vi "OpenCVFaceDetection_NewMat.vi"(8 "ErrorIn":errorcluster, 10 "CmdData":variant, 11 "OpenCVFaceDetectionIn":refnum<class>) -> (0 "ErrorOut":errorcluster, 2 "ReplyData":variant, 3 "OpenCVFaceDetectionOut":refnum<class>, 4 "Exit":bool)   [LabVIEW 2021, in "OpenCVFaceDetection.lvclass"]
uses:
  OpenCVFaceDetection.lvclass
  OpenCVFaceDetection_UiCallBackEvents.ctl
  OpenCVFaceDetection.lvclass/OpenCVFaceDetection.ctl
  9f33c80a-1a62-43e8-9ad8-ec198e7f1f80.vi
  System.Drawing
  C:/Localdata/Projects/TriekselSoft/TriekselsoftApplicationFramework/Source/.Externals/Library_EmguCV/Emgu.CV.Platform.NetStandard.dll
  .Externals/Library_EmguCV/Emgu.CV.Platform.NetStandard.dll
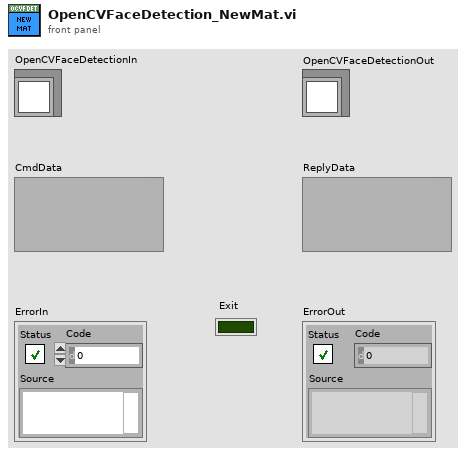
[diagram p1: front panel]
types:
  T1 = typedef "OpenCVFaceDetection.lvclass/OpenCVFaceDetection_UiCallBackEvents.ctl" = enum16{"Default", "PersistentDataUpdated", "NewPicture", "Worker 1: Do Something"}
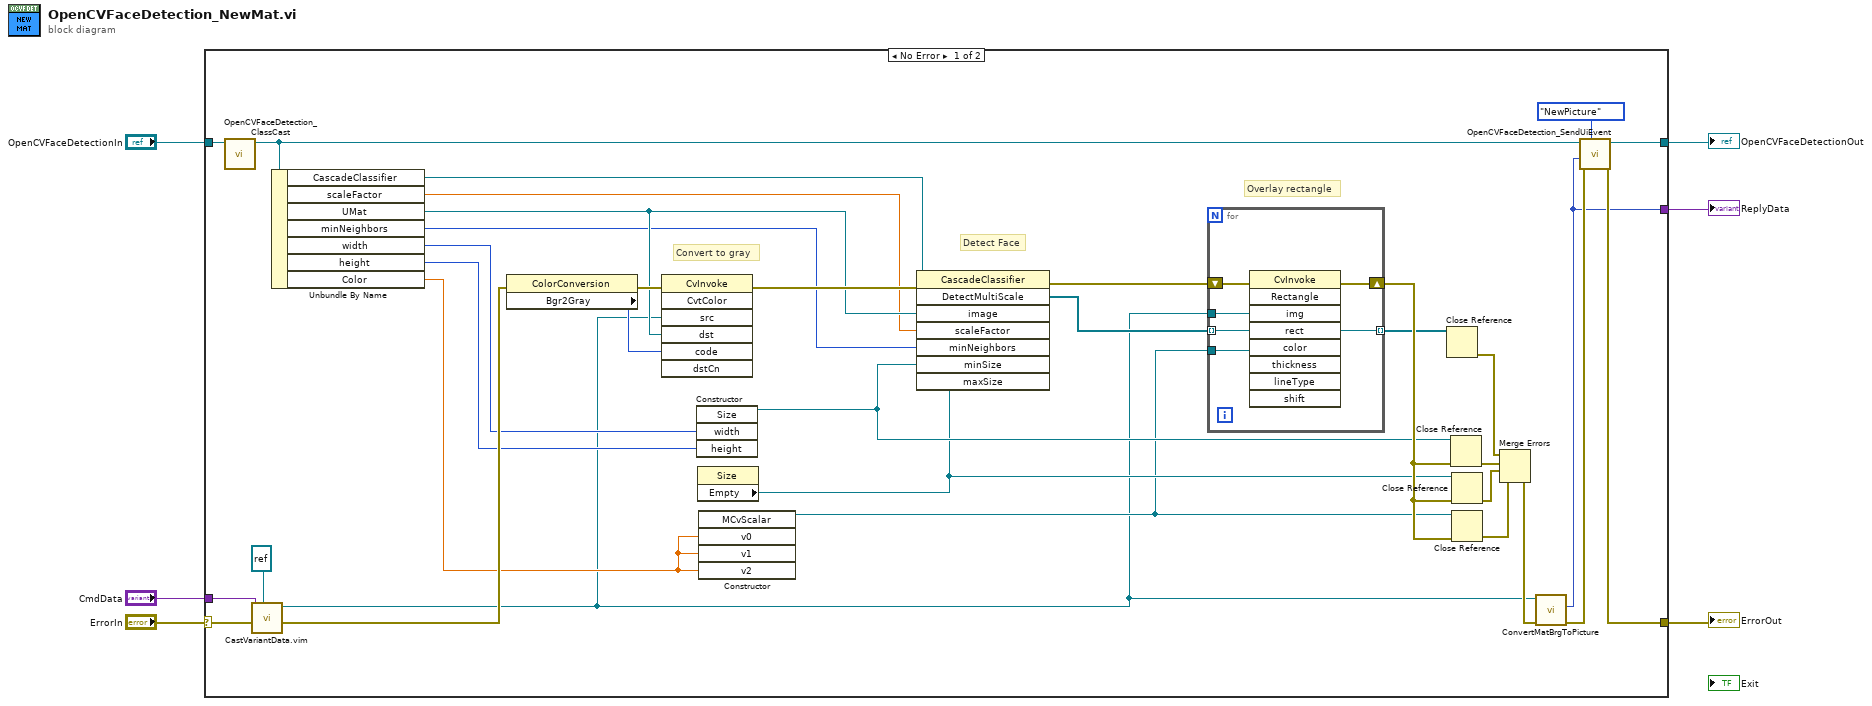
[diagram p0: block diagram]
diagram:
  n1 = case shown="No Error" "ErrorIn" {
    selector: "ErrorIn" -> [w40 w48]
    tunnel: [w29 w48] -> w5
    tunnel: [w9 w47] -> w3
    tunnel: "CmdData" -> [w26 w47]
    tunnel: "OpenCVFaceDetectionIn" -> [w27 w46]
    tunnel: [w10 w46] -> w1
    frame No Error {
      # "Overlay rectangle"
      # "Detect Face"
      # "Convert to gray"
      n2 = call "OpenCVFaceDetection_ClassCast.vi"("OpenCVFaceDetectionIn"=w27) -> ("OpenCVFaceDetectionOut"=w20:refnum<class "OpenCVFaceDetection.lvclass">)  [unwired: 10 in]
      n3 = call "CastVariantData.vim"("Type"=refnum<k24> refnum ("CvMat"), "ErrorIn"=w40, "DataIn"=w26) -> ("ErrorOut"=w37:errorcluster, "DataOut"=w11:refnum<k24>)  [unwired: 7 in]
      n4 = Unbundle By Name(w20) -> ("CascadeClassifier"=w21:refnum<k24>, "scaleFactor"=w19:dbl, "UMat"=w22:refnum<k24>, "minNeighbors"=w18:i32, "width"=w17:i32, "height"=w16:i32, "Color"=w15:dbl)
      n5 = property class="ColorConversion"(error in=w37) -> (error out=w38:errorcluster, "Bgr2Gray"=w24:i32)  [unwired: 1 in, 1 out]
      n6 = invoke class="CvInvoke" method="CvtColor"(error in=w38, "src"=w11, "dst"=w22, "code"=w24) -> (error out=w39:errorcluster)  [unwired: 3 in, 6 out]
      n7 = constructor class="Size"("width"=w17, "height"=w16) -> (reference out=w14:refnum<k24>)  [unwired: 3 in, 4 out]
      n8 = property class="Size"() -> ("Empty"=w13:refnum<k24>)  [unwired: 2 in, 2 out]
      n9 = constructor class="MCvScalar"("v0"=w15, "v1"=w15, "v2"=w15) -> (reference out=w12:refnum<k24>)  [unwired: 3 in, 5 out]
      n10 = invoke class="CascadeClassifier" method="DetectMultiScale"(reference=w21, error in=w39, "image"=w22, "scaleFactor"=w19, "minNeighbors"=w18, "minSize"=w14, "maxSize"=w13) -> (error out=w36:errorcluster, "DetectMultiScale"=w23:refnum<k24>[])  [unwired: 1 in, 6 out]
      n11 = for {
        tunnel: w23 -> [w41] mode=indexing
        tunnel: w12 -> [w43]
        tunnel: w11 -> [w42]
        shift-right: [w45] -> w35
        shift-left: w36 -> [w44]
        tunnel: [w41] -> w7 mode=indexing
        n12 = invoke class="CvInvoke" method="Rectangle"(error in=w44, "img"=w42, "rect"=w41, "color"=w43) -> (error out=w45:errorcluster)  [unwired: 5 in, 8 out]
      }
      n13 = Close Reference(reference=w7) -> (error out=w28:errorcluster)  [unwired: 1 in]
      n14 = Close Reference(reference=w14, error in (no error)=w35) -> (error out=w34:errorcluster)
      n15 = Close Reference(reference=w13, error in (no error)=w35) -> (error out=w33:errorcluster)
      n16 = Close Reference(reference=w12, error in (no error)=w35) -> (error out=w32:errorcluster)
      n17 = Merge Errors(w28, w34, w33, w32) -> (w31:errorcluster)
      n18 = call "ConvertMatBrgToPicture.vi"("ErrorIn"=w31, "CvMatIn"=w11) -> ("ErrorOut"=w30:errorcluster, "NewPicture"=w9:picture)  [unwired: 7 in, 1 out]
      n19 = call "OpenCVFaceDetection_SendUiEvent.vi"("UiEventNames"=OpenCVFaceDetection_UiCallBackEvents."NewPicture", "ErrorIn"=w30, "Data"=w9, "OpenCVFaceDetectionIn"=w20) -> ("ErrorOut"=w29:errorcluster, "OpenCVFaceDetectionOut"=w10:refnum<class "OpenCVFaceDetection.lvclass">)  [unwired: 6 in]
    }
    frame Error {
    }
  }
  "ErrorOut" <- w5
  "OpenCVFaceDetectionOut" <- w1
  "ReplyData" <- w3
